vi "Fetch Calibration Points.vi"(8 "error in (no error)":errorcluster, 10 "SQL Query":string, 11 "Refnum in":T1) -> (0 "error out":errorcluster, 2 "Results":string[][](array[string]), 3 "Refnum out":T1)   [LabVIEW 2026, in "Database.lvlib"]
uses:
  <vilib>/addons/database/Connection.llb/Conn ObjectReference.ctl
  <vilib>/addons/database/Connection.llb/Conn Execute.vi
  Database.lvlib
  <vilib>/addons/database/NI_Database_API.lvlib
  <vilib>/addons/database/Recordset.llb/Rec Fetch Recordset Data (R).vi
  <vilib>/addons/database/_DB Variant To Data/Database Variant To Data.xnode
  <vilib>/addons/database/Recordset.llb/Rec Destroy - Connection.vi
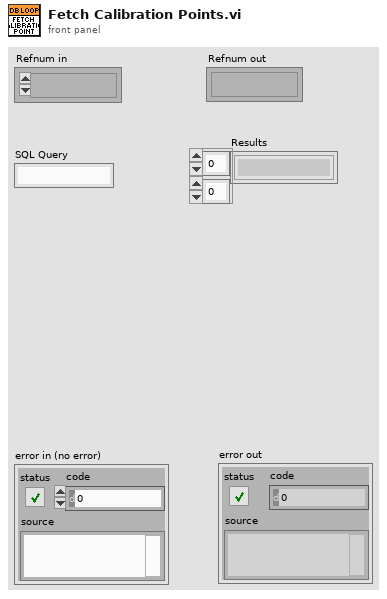
[diagram p1: front panel]
types:
  T1 = typedef "NI_Database_API.lvlib/Conn ObjectReference.ctl" = refnum<k1>
  T2 = typedef "NI_Database_API.lvlib/Rec ObjectReference.ctl" = refnum<k1>
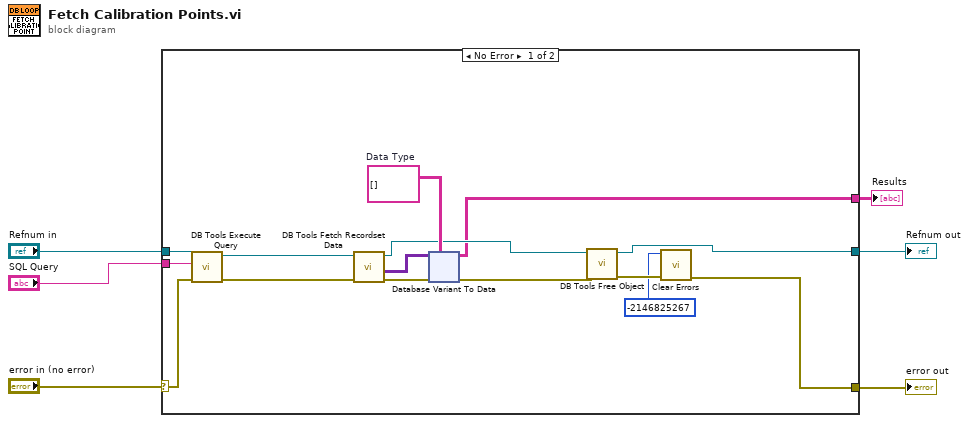
[diagram p0: block diagram]
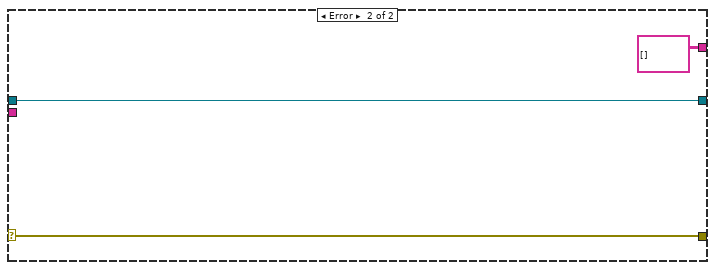
[diagram p2: hidden frame]
diagram:
  n1 = case shown="No Error" "error in (no error)" {
    selector: "error in (no error)" -> [w15 w68]
    tunnel: [w21 w67] -> w6
    tunnel: [w20 w68] -> w5
    tunnel: "SQL Query" -> [w17 _]
    tunnel: "Refnum in" -> [w16 w67]
    tunnel: [w7 string[][] [] ("data")] -> w1
    frame No Error {
      w10 = string[][] []  # Data Type
      n2 = call-poly <vilib>:"DB Tools Execute Query.vi"("error in (no error)"=w15, "SQL query"=w17, "connection reference"=w16) -> ("error out"=w13:errorcluster, "recordset reference"=w14:T2)  [unwired: 5 in]
      n3 = call-poly <vilib>:"DB Tools Fetch Recordset Data.vi"("error in (no error)"=w13, "recordset reference"=w14) -> ("error out"=w12:errorcluster, "recordset data"=w11:variant[][], "recordset reference out"=w8:T2)  [unwired: 3 in]
      n4 = xnode "Database Variant To Data"("database variant"=w11, "error in (no error)"=w12, "type"=w10) -> ("data"=w7:string[][], "error out"=w9:errorcluster)
      n5 = call-poly <vilib>:"DB Tools Free Object.vi"("error in (no error)"=w9, "recordset reference"=w8) -> ("error out"=w19:errorcluster, "connection reference"=w21:T1)  [unwired: 8 in]
      n6 = call <vilib>:"Clear Errors.vi"("error in (no error)"=w19, "specific error code to clear (0: all)"=-2146825267) -> ("error out"=w20:errorcluster)  [unwired: 4 in, 1 out]
    }
    frame Error {
    }
  }
  "Refnum out" <- w6
  "error out" <- w5
  "Results" <- w1
